vi "ScanBoxB_Loopready.vi"(11 "YTESTER测试数据":T1={"Socket(From1)"=1, "SN"=refnum, "StopFlagRef"=refnum, "YT System Queue"=refnum}) -> (3 "YTESTER结论":T2)   [LabVIEW 2017]
doc: "VIDescription="
uses:
  YtCommon.lvlibp/yt`Step StepBaseInput.ctl
  YtCommon.lvlibp/yt`Step StepResult.ctl
  YtCommon.lvlibp/yt`Step TestData.ctl
  YtCommon.lvlibp/yt`Step System Queue.ctl
  Step`s VIs/YYLLGeneric/variable_W.ctl
  YtCommon.lvlibp/yt`Data-Ytester Type Data.ctl
  YtCommon.lvlibp
panel:
  out "SN out":string
  in  "YTESTER开放参数":T4={"YTESTER_BaseInput"={"isTest"=TRUE, "isSkip"=FALSE, "StepName"="ScanBoxB请扫码！", "OnPass"=enum."Next", "OnFail"=enum."Terminate", "ReTestNumber"=0.0}, "扫码项名称"="SN：", "扫码长度"=0, "扫码项开头匹配"="", "Smart预处理"=[], "扫码到变量(自定义建议#开头)"="不到变量", "类回车确认"=TRUE, "Color FG"=6416282, "设置为主SN"=FALSE, "Poztion"=enum."中"}
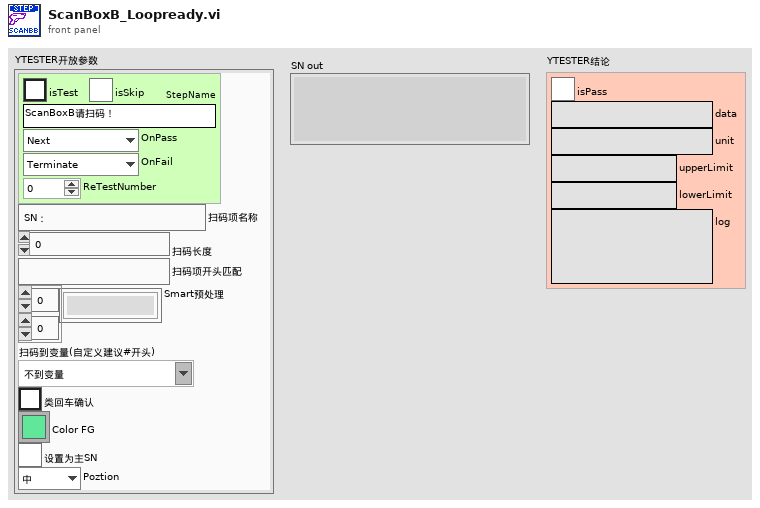
[diagram p1: front panel]
types:
  T1 = typedef "YtCommon.lvlibp/yt`Step TestData.ctl" = cluster{"Socket(From1)":i32, "SN":refnum<notifier>, "StopFlagRef":refnum<notifier>, "YT System Queue":refnum<queue>}
  T2 = typedef "YtCommon.lvlibp/yt`Step StepResult.ctl" = cluster{"isPass":bool, "data":string, "unit":string, "upperLimit":string, "lowerLimit":string, "log":string}
  T3 = typedef "YtCommon.lvlibp/yt`Step StepBaseInput.ctl" = cluster{"isTest":bool, "isSkip":bool, "StepName":string, "OnPass":enum16{"Next", "ToOVER", "Terminate"}, "OnFail":enum16{"Next", "ToOVER", "Terminate"}, "ReTestNumber":dbl}
  T4 = cluster{"YTESTER_BaseInput":T3, "扫码项名称":string, "扫码长度":i32, "扫码项开头匹配":string, "Smart预处理":string[][], "扫码到变量(自定义建议#开头)":string, "类回车确认":bool, "Color FG":u32, "设置为主SN":bool, "Poztion":enum16{"↖", "↑", "↗", "←", "中", "→", "↙", "↓", "↘"}}
  T5 = enum16{"↖", "↑", "↗", "←", "中", "→", "↙", "↓", "↘"}
  T6 = typedef "variable_W.ctl" = cluster{"YT_TYPE":T7, "TypeData":string[], "Tips":string}
  T7 = typedef "YtCommon.lvlibp/yt`Data-Ytester Type Data.ctl" = enum16{"NULL", "NUM", "BOOL", "TXT", "ENUM", "TIME", "PATH", "VISA", "COMBO", "ColorBox", "RadioBtn", "Array_NUM", "Array_BOOL", "Array_TXT", "Array_ENUM", "Array_PATH", "Array_COMBO"}
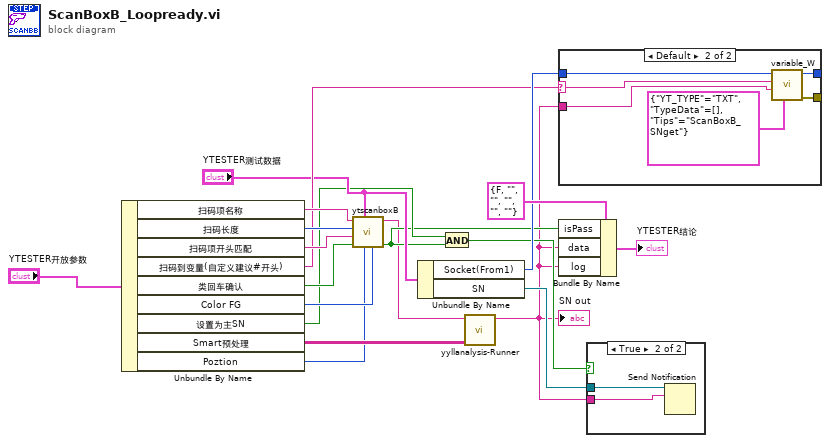
[diagram p0: block diagram]
diagram:
  n1 = Unbundle By Name("YTESTER开放参数") -> ("扫码项名称"=w16:string, "扫码长度"=w15:i32, "扫码项开头匹配"=w14:string, "扫码到变量(自定义建议#开头)"=w11:string, "类回车确认"=w13:bool, "Color FG"=w9:u32, "设置为主SN"=w6:bool, "Smart预处理"=w2:string[][], "Poztion"=w1:T5)
  n2 = call "ytscanboxB.vi"("Color FG"=w9, "Poztion"=w1, "YTESTER测试数据"="YTESTER测试数据", "类回车确认"=w13, "扫码项开头匹配"=w14, "扫码长度"=w15, "扫码项名称"=w16) -> ("pass?"=w5:bool, "SN out"=w4:string)  [unwired: 3 in]
  n3 = Unbundle By Name("YTESTER测试数据") -> ("Socket(From1)"=w12:i32, "SN"=w8:refnum<notifier>)
  n4 = And(x=w6, y=w5) -> (x .and. y?=w7:bool)
  n5 = call "yyllanalysis-Runner.vi"("inputs"=w2, "String in"=w4) -> ("String out"=w3:string)  [unwired: 8 in, 1 out]
  "SN out" <- w3
  n6 = case shown="Default" w11 {
    selector: w11 -> [_ w25]
    tunnel: w12 -> [w20 w26]
    tunnel: [w20 w23] -> _
    tunnel: w3 -> [_ w22]
    tunnel: [_ w21] -> _
    frame "不到变量" {
    }
    frame Default {
      n7 = call "variable_W.vi"("附加的Information"=T6 {"YT_TYPE"=enum."TXT", "TypeData"=[], "Tips"="ScanBoxB_SNget"}, "待写入池的输入控件"=w22, "待写入池变量名称"=w25, "函数池名称 in"=w26) -> ("error out"=w21:errorcluster, "函数池名称 out"=w23:i32)  [unwired: 5 in, 1 out]
    }
  }
  n8 = Bundle By Name(cluster=T2 {"isPass"=FALSE, "data"="", "unit"="", "upperLimit"="", "lowerLimit"="", "log"=""} ("Result"), "isPass"=w5, "data"=w3, "log"=w3) -> (→"YTESTER结论":T2)
  n9 = case shown="True" w7 {
    tunnel: w8 -> [_ w28]
    tunnel: w3 -> [_ w27]
    frame False {
    }
    frame True {
      n10 = Send Notification(notification=w27, notifier=w28) -> ()  [unwired: 1 in, 2 out]
    }
  }
